vi "Blynk LED.vi"(8 "error in (no error)":errorcluster, 9 "value":string, 10 "pin":string, 11 "connection":refnum<k5>) -> (0 "error out":errorcluster, 3 "connection out":refnum<k5>)   [LabVIEW 2014]
uses:
  utilities/MsgType.ctl
panel:
  out "data out":string
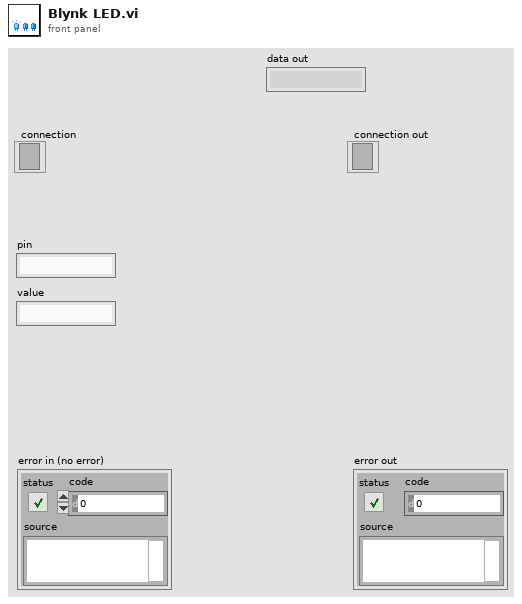
[diagram p1: front panel]
types:
  T1 = typedef "MsgType.ctl" = enum8{"RSP", "REGISTER", "LOGIN", "SAVE_PROF", "LOAD_PROF", "GET_TOKEN", "PING", "ACTIVATE", "DEACTIVATE", "REFRESH", "UNDEFINED0", "UNDEFINED1", "TWEET", "EMAIL", "NOTIFY", "BRIDGE", "UNDEFINED2", "UNDEFINED3", "UNDEFINED4", "UNDEFINED5", "HW"}
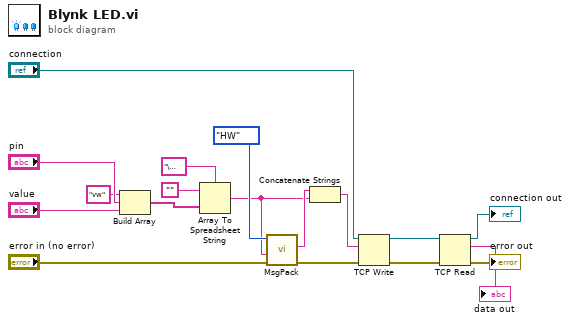
[diagram p0: block diagram]
diagram:
  n1 = Build Array("vw" ("element"), "pin", "value") -> (w10:string[])
  n2 = Array To Spreadsheet String(delimiter (Tab)="\u0000", array=w10, 3:"") -> (spreadsheet string=w14:string)
  n3 = call "MsgPack.vi"("error in"="error in (no error)", "msg"=w14, "msg_type"=MsgType."HW") -> ("error out"=w7:errorcluster, "msg_data"=w17:string)  [unwired: 7 in]
  n4 = Concatenate Strings(w17, w14) -> (w18:string)
  n5 = TCP Write(connection ID="connection", data in=w18, error in (no error)=w7) -> (connection ID out=w5:refnum<k5>, error out=w3:errorcluster)  [unwired: 1 in, 1 out]
  n6 = TCP Read(connection ID=w5, error in (no error)=w3) -> (connection ID out=→"connection out":refnum<k5>, data out=→"data out":string, error out=→"error out":errorcluster)  [unwired: 3 in]
